vi "GetClass.vi"(8 "error in (no error)":errorcluster, 11 "Pulseblaster in":refnum<class "Slave_Pulseblaster.lvclass">) -> (0 "error out":errorcluster, 2 "Device Class":string="Device->Slave_Pulseblaster", 3 "Pulseblaster out":refnum<class "Slave_Pulseblaster.lvclass">)   [LabVIEW 2013, in "Slave_Pulseblaster.lvclass"]
uses:
  Slave_Pulseblaster.lvclass
  Device/Device.lvclass
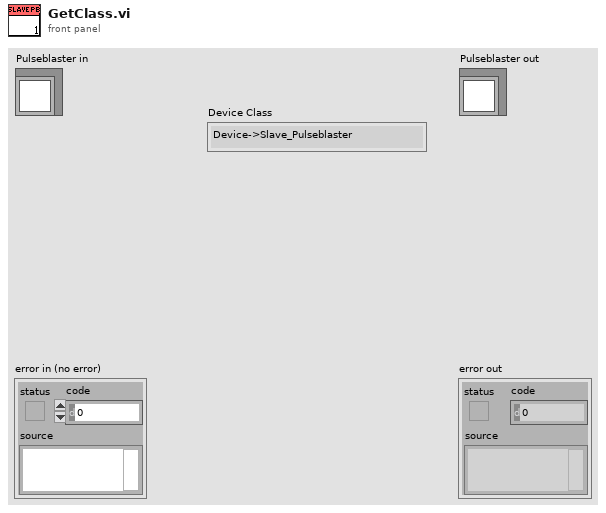
[diagram p1: front panel]
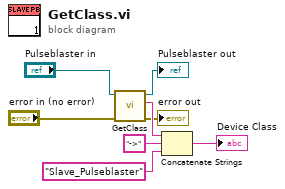
[diagram p0: block diagram]
diagram:
  n1 = call-parent "GetClass.vi"("error in (no error)"="error in (no error)", "Device in"="Pulseblaster in") -> ("error out"=→"error out":errorcluster, "Device Class"=w6:string, "Device out"=→"Pulseblaster out":refnum<class "Slave_Pulseblaster.lvclass">)  [unwired: 7 in]
  n2 = Concatenate Strings(w6, "->" ("string"), "Slave_Pulseblaster") -> (→"Device Class":string)
